vi "rydberg_write_synth_channel.vi"(8 "Channel #":i32, 9 "Channel Active":bool, 10 "Channel Parameters":T1={"Voltage (Amp.) "=0.0, "Frequency (MHz)"=0.0, "Phase (deg)"=0.0, "Nickname"="Channel 0 D"}) -> (2 "Command":string)   [LabVIEW 2016]
uses:
  Controls/Synth_409b/synth_channel.ctl
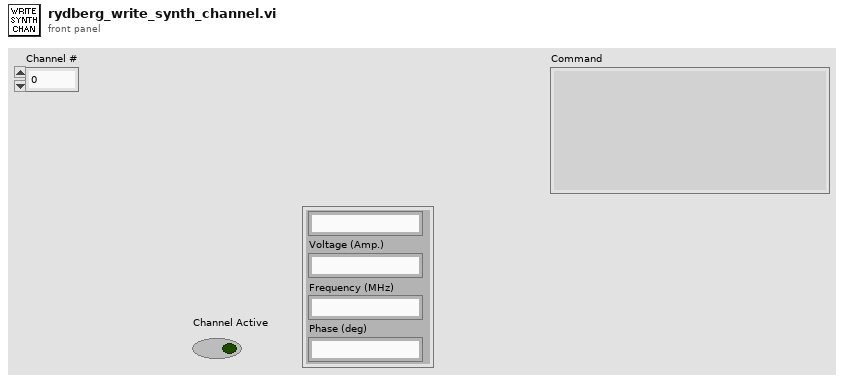
[diagram p1: front panel]
types:
  T1 = typedef "synth_channel.ctl" = cluster{"Voltage (Amp.) ":dbl, "Frequency (MHz)":dbl, "Phase (deg)":dbl, "Nickname":string}
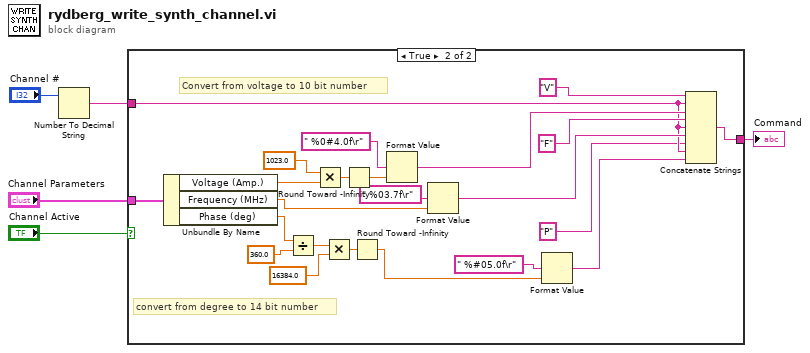
[diagram p0: block diagram]
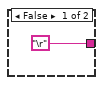
[diagram p2: hidden frame]
diagram:
  n1 = Number To Decimal String(number="Channel #") -> (decimal integer string=w3:string)  [unwired: 1 in]
  n2 = case shown="True" "Channel Active" {
    tunnel: "Channel Parameters" -> [_ w29]
    tunnel: w3 -> [_ w13]
    tunnel: ["\r" w8] -> w2
    frame False {
    }
    frame True {
      # "convert from degree to 14 bit number"
      # "Convert from voltage to 10 bit number"
      n3 = Unbundle By Name(w29) -> ("Voltage (Amp.)"=w28:dbl, "Frequency (MHz)"=w7:dbl, "Phase (deg)"=w25:dbl)
      n4 = Divide(x=w25, y=360.0) -> (x/y=w23:dbl)
      n5 = Multiply(x=1023.0, y=w28) -> (x*y=w26:dbl)
      n6 = Multiply(x=w23, y=16384.0) -> (x*y=w21:dbl)
      n7 = Round Toward -Infinity(1:w26) -> (0:w20:dbl)
      n8 = Round Toward -Infinity(1:w21) -> (0:w11:dbl)
      n9 = Format Value(format string=" %0#4.0f\r", value (0)=w20) -> (output string=w17:string)  [unwired: 1 in]
      n10 = Format Value(format string=" %03.7f\r", value (0)=w7) -> (output string=w14:string)  [unwired: 1 in]
      n11 = Format Value(format string=" %#05.0f\r", value (0)=w11) -> (output string=w9:string)  [unwired: 1 in]
      n12 = Concatenate Strings("V", w13, w17, "F" ("string"), w13, w14, "P" ("string"), w13, w9) -> (w8:string)
    }
  }
  "Command" <- w2
